vi "FTW-JSON-Core-ElementType.vi"(0 "JSON Element":i64 format="%016x", 11 "error in":errorcluster) -> (4 "JSON Element out":i64 format="%016x", 6 "JSON Type":T1=enum."undefined", 15 "error out":errorcluster)   [LabVIEW 2013]
uses:
  FTW-JSON-Type.ctl
panel:
  # "Inputs"
  # "Outputs"
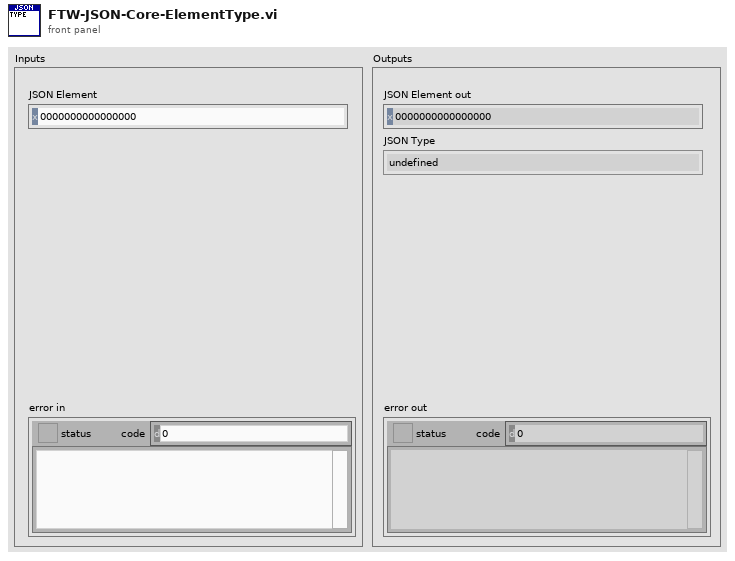
[diagram p1: front panel]
types:
  T1 = typedef "FTW-JSON-Type.ctl" = enum16{"Object", "Array", "String", "Integer", "Floating Point", "true", "false", "null", "undefined"}
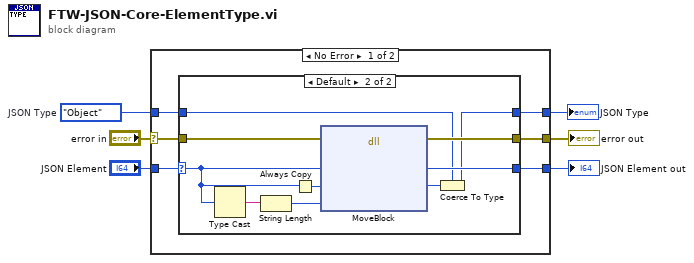
[diagram p0: block diagram]
diagram:
  w2 = FTW-JSON-Type."Object"  # JSON Type
  n1 = case shown="No Error" "error in" {
    selector: "error in" -> [w11 w28]
    tunnel: [w10 w28] -> w6
    tunnel: [w9 w27] -> w5
    tunnel: "JSON Element" -> [w12 w27]
    tunnel: w2 -> [w8 w26]
    tunnel: [w7 w26] -> w1
    frame No Error {
      n2 = case shown="Default" w12 {
        selector: w12 -> [w14 w17]
        tunnel: w11 -> [w13 w25]
        tunnel: [w13 w24] -> w10
        tunnel: [w14 w23] -> w9
        tunnel: [w15 w19] -> w7
        tunnel: w8 -> [w15 w16]
        frame 0 {
        }
        frame Default {
          n3 = Type Cast(x=w17) -> (*(type *) &x=w22:string)  [unwired: 1 in]
          n4 = String Length(string=w22) -> (length=w21:i32)
          n5 = Always Copy(1:w17) -> (0:w18:i64)
          n6 = dll-call lib="LabVIEW" fn="MoveBlock"(error in=w25, "Source Pointer"=w17, "Destination Buffer"=w18, "Buffer Size"=w21) -> (error out=w24:errorcluster, "Source Pointer"=w23:i64, "Destination Buffer"=w20:i64)  [unwired: 4 in, 1 out]
          n7 = Coerce To Type(0:w20, 1:w16) -> (2:w19:T1)
        }
      }
    }
    frame Error {
    }
  }
  "error out" <- w6
  "JSON Element out" <- w5
  "JSON Type" <- w1
